vi "GetPhaseNumber.vi"(10 "Loop Counter":i32, 11 "Phase(-1, all) in":i32) -> (3 "Phase(-1, all) out":i32)   [LabVIEW 2018, in "AcPwrPlugins.lvlib" / "AcPwrBase.lvclass"]
uses:
  AcPwrBaseClass/AcPwrBase.lvclass
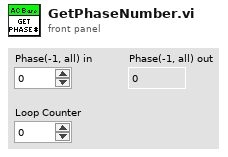
[diagram p1: front panel]
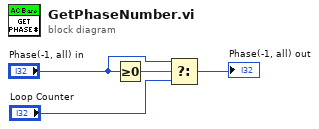
[diagram p0: block diagram]
diagram:
  n1 = Greater Or Equal To 0?(x="Phase(-1, all) in") -> (x >= 0?=w2:bool)
  n2 = Select(t="Phase(-1, all) in", s=w2, f="Loop Counter") -> (s? t:f=→"Phase(-1, all) out":i32)
